vi "CTI_AOTF_set_params.vi"(1 "frequency":i32[](array[numeric]), 2 "Numeric":i32, 3 "error IO":errorcluster, 4 "Array":bool[](array[boolean]), 5 "amplitude":i16[](array[numeric]), 6 "CTI AOTF-Controller":refnum<visa-resource-name>) -> (0 "error out":errorcluster)   [LabVIEW 2013]
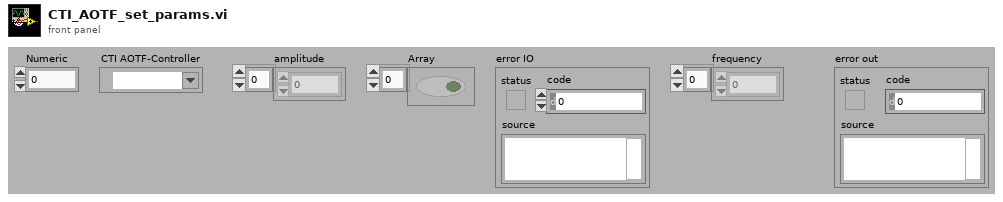
[diagram p1: front panel]
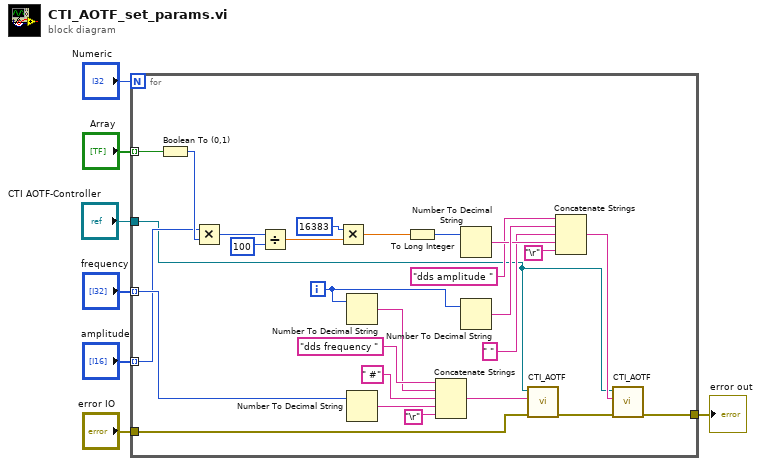
[diagram p0: block diagram]
diagram:
  n1 = for {
    N: "Numeric" -> [_]
    tunnel: "frequency" -> [w27] mode=indexing
    tunnel: "amplitude" -> [w16] mode=indexing
    tunnel: "error IO" -> [w34]
    tunnel: [w12] -> w3
    tunnel: "Array" -> [w9] mode=indexing
    tunnel: "CTI AOTF-Controller" -> [w8]
    i -> [w10]
    n2 = Boolean To (0,1)(Boolean=w9) -> (0, 1=w17:i16)
    n3 = Multiply(x=w16, y=w17) -> (x*y=w15:i16)
    n4 = Divide(x=w15, y=100) -> (x/y=w24:dbl)
    n5 = Multiply(x=16383, y=w24) -> (x*y=w22:dbl)
    n6 = Number To Decimal String(number=w10) -> (decimal integer string=w32:string)  [unwired: 1 out]
    n7 = Number To Decimal String(number=w27) -> (decimal integer string=w30:string)  [unwired: 1 out]
    n8 = To Long Integer(number=w22) -> (32bit integer=w18:i32)
    n9 = Concatenate Strings("dds frequency " ("string"), w32, " #" ("string"), w30, "\r") -> (w28:string)
    n10 = Number To Decimal String(number=w18) -> (decimal integer string=w20:string)  [unwired: 1 out]
    n11 = Number To Decimal String(number=w10) -> (decimal integer string=w26:string)  [unwired: 1 out]
    n12 = call "CTI_AOTF.vi"("error in"=w34, "String"=w28, "VISA resource name 2"=w8) -> ("error out"=w13:errorcluster)  [unwired: 7 in, 1 out]
    n13 = Concatenate Strings("dds amplitude " ("string"), w26, " " ("string"), w20, "\r") -> (w11:string)
    n14 = call "CTI_AOTF.vi"("error in"=w13, "String"=w11, "VISA resource name 2"=w8) -> ("error out"=w12:errorcluster)  [unwired: 7 in, 1 out]
  }
  "error out" <- w3
